vi "zc_tg.vi"(0 "action":string, 1 "LabVIEW Web Service Request":refnum<class "Web Request.lvclass"> caption="LabVIEW Web服务请求", 2 "zhriqi":string, 3 "sp_yijian":string, 4 "key":string, 5 "id":string, 7 "zc_luodi_num":string, 8 "sp_shuoming":string, 9 "didian":string, 11 "jsren":string, 13 "shuoming":string, 14 "lc_num":string) -> (15 "error":errorcluster)   [LabVIEW 2017]
uses:
  <vilib>/wsapi/Web Request.lvclass
panel:
  in  "error 3":errorcluster={"status"=TRUE, "code"=255, "source"="当前资产不是“领用”状态！"} caption="error"
  out "postdata":string caption="post数据"
  out "error out":errorcluster caption="错误输出"
  # "Web服务请求输入接线端用于调用“Web服务”选板的VI。除非不需要访问该选板，否则不要在连线板上删除这个输入接线端。"
  # "添加至连线板的每一个其他输入控件，在URL中对应于一个输入。如需在接线端模式输出（默认设置）下包含显示控件，则该显示控件必须与连线板相连。"
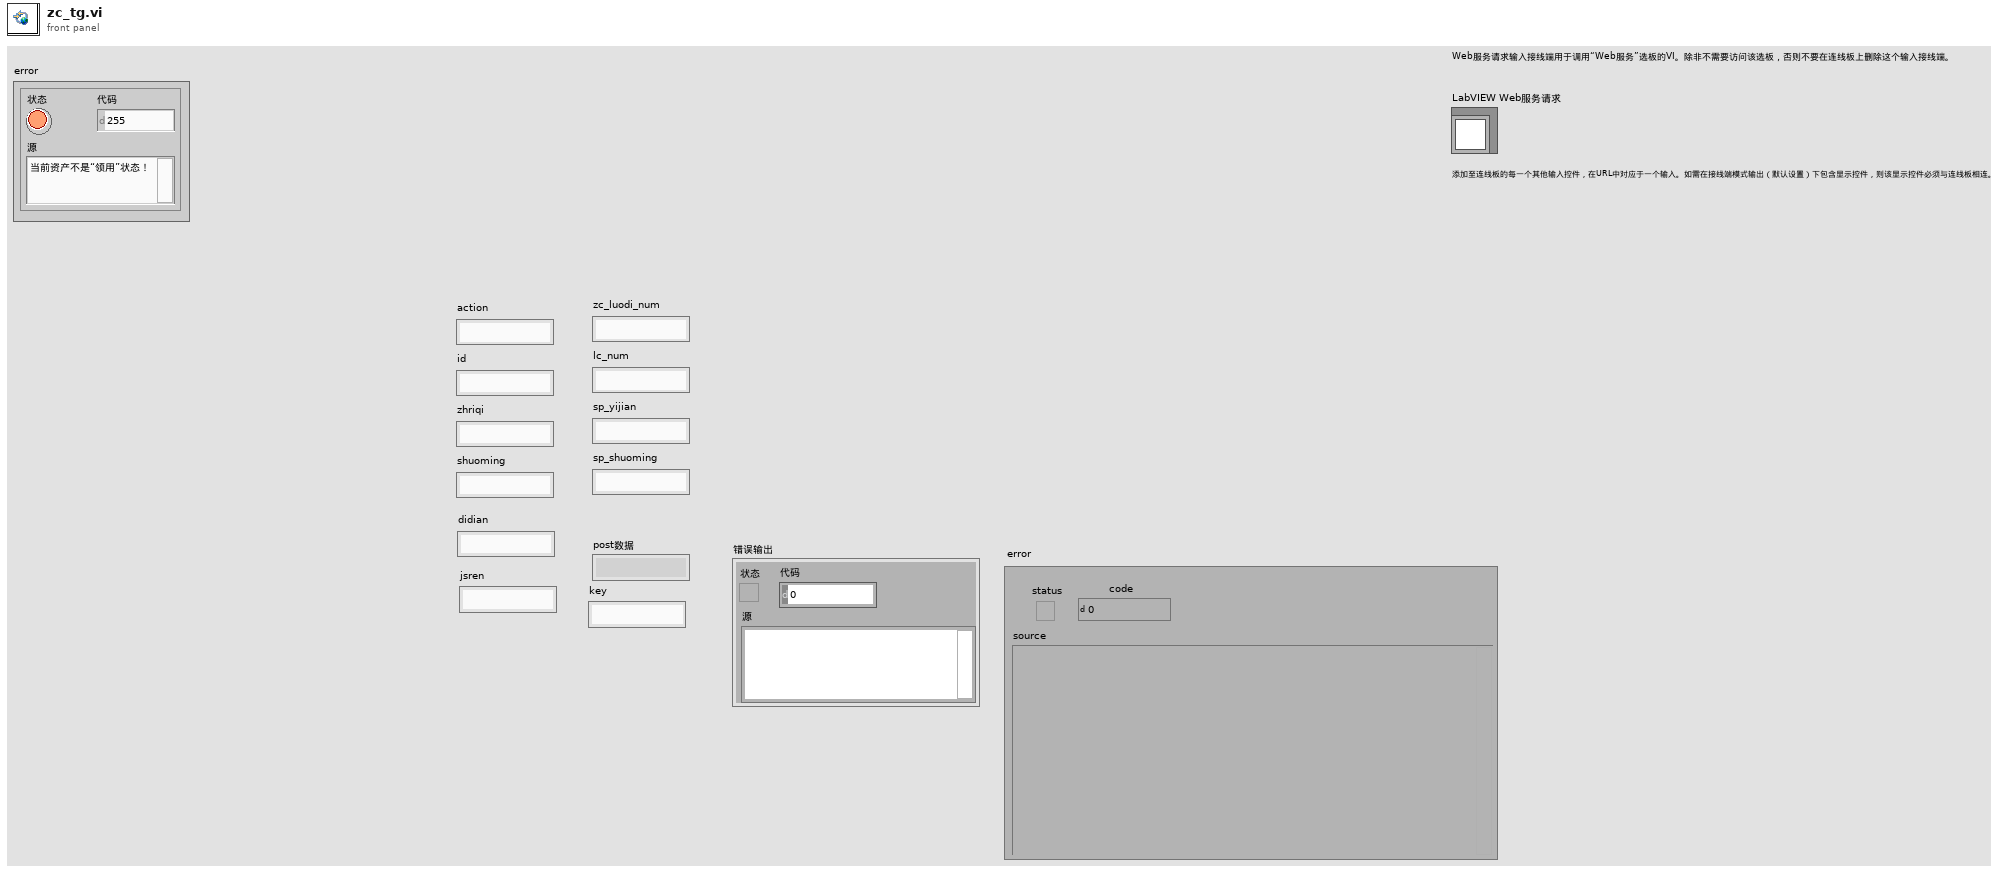
[diagram p1: front panel]
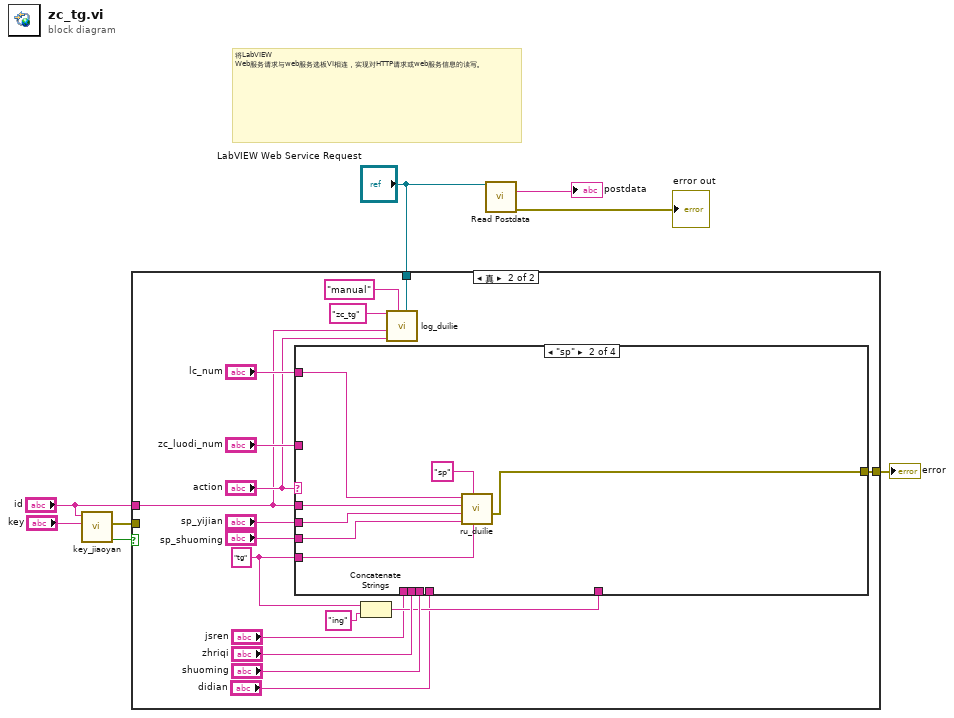
[diagram p0: block diagram]
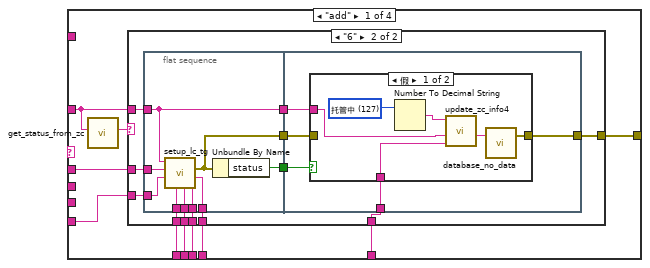
[diagram p3: hidden frame]
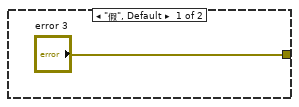
[diagram p4: hidden frame]
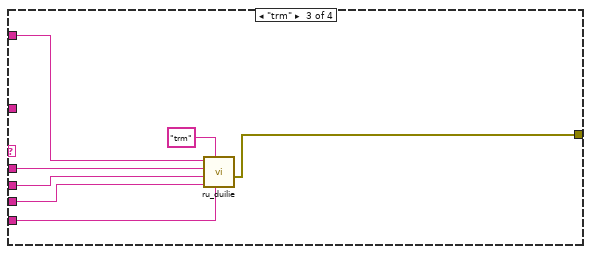
[diagram p6: hidden frame]
diagram:
  # "将LabVIEW Web服务请求与web服务选板VI相连，实现对HTTP请求或web服务信息的读写。"
  n1 = call "key_jiaoyan.vi"("key_client"="key", "gonghao"="id") -> ("jy"=w2:bool, "error"=w1:errorcluster)  [unwired: 8 in]
  n2 = case shown="真" w2 {
    tunnel: [w9 w20] -> w7
    tunnel: "LabVIEW Web Service Request" -> [_ w12]
    tunnel: "id" -> [_ w10]
    tunnel: w1 -> [w9 _]
    frame False {
    }
    frame True {
      w18 = "tg" ("yw")
      n3 = Concatenate Strings(w18, "ing" ("字符串")) -> (w17:string)
      n4 = case shown="\"sp\"" "action" {
        tunnel: w10 -> [w34 w76 w83 _]
        tunnel: "zc_luodi_num" -> [w28 _ _ _]
        tunnel: "sp_yijian" -> [_ w74 w81 _]
        tunnel: "sp_shuoming" -> [_ w73 w80 _]
        tunnel: "zhriqi" -> [w36 _ _ _]
        tunnel: "shuoming" -> [w35 _ _ _]
        tunnel: w18 -> [w33 w72 w79 _]
        tunnel: "lc_num" -> [_ w75 w82 _]
        tunnel: [w32 w71 w78 _] -> w20
        tunnel: w17 -> [w31 _ _ _]
        tunnel: "jsren" -> [w30 _ _ _]
        tunnel: "didian" -> [w29 _ _ _]
        frame "add" {
          n5 = call "get_status_from_zc.vi"("zc_luodi_num"=w28) -> ("status"=w27:string)  [unwired: 9 in, 1 out]
          n6 = case shown="\"6\"" w27 {
            tunnel: w36 -> [_ w48]
            tunnel: w35 -> [_ w47]
            tunnel: w34 -> [_ w46]
            tunnel: w33 -> [_ w45]
            tunnel: ["error 3" w44] -> w32
            tunnel: w31 -> [_ w43]
            tunnel: w30 -> [_ w42]
            tunnel: w29 -> [_ w41]
            tunnel: w28 -> [_ w40]
            frame "假", Default {
            }
            frame "6" {
              n7 = flat-sequence {
                tunnel: w48 -> [w54]
                tunnel: w47 -> [w53]
                tunnel: w40 -> [w58]
                tunnel: w46 -> [w56]
                tunnel: w45 -> [w57]
                tunnel: [w58] -> w49
                tunnel: w42 -> [w55]
                tunnel: w41 -> [w52]
                tunnel: [w51] -> w39
                tunnel: [w50] -> w38
                tunnel: w49 -> [w62]
                tunnel: [w63] -> w44
                tunnel: w43 -> [w61]
                tunnel: w39 -> [w60]
                tunnel: w38 -> [w59]
                frame #0 {
                  n8 = call "setup_lc_tg.vi"("shuoming"=w53, "didian"=w52, "zhriqi"=w54, "jsren"=w55, "yw"=w57, "id"=w56, "zc_luodi_num"=w58) -> ("error"=w50:errorcluster)  [unwired: 4 in]
                  n9 = Unbundle By Name(w50) -> ("status"=w51:bool)
                }
                frame #1 {
                  n10 = case shown="假" w60 {
                    tunnel: [w68 w70] -> w63
                    tunnel: w62 -> [w66 _]
                    tunnel: w61 -> [w65 _]
                    tunnel: w59 -> [_ w70]
                    frame False {
                      w67 = u8 127 items=["待验收"=1, "无需验收"=2, "验收不合格"=3, "待入库"=4, "入库"=5, "领用"=6, "借用"=7, "托管"=8, "接管"=9, "退出"=10, "出库在用"=11, "盘亏"=12, "出售"=13, "报废"=14, "领用中"=120, "退库中"=121, "借用中"=122, "归还中"=123, "转移中"=124, "调拨中"=125, "借调中"=126, "托管中"=127, "终止托管中"=128, "退出中"=129, "处置中"=130] ("状态选择器")
                      n11 = Number To Decimal String(number=w67) -> (decimal integer string=w64:string)  [unwired: 1 in]
                      n12 = call "update_zc_info4.vi"("ywxinxi"=w65, "number"=w66, "status"=w64) -> ("data_str"=w69:string)  [unwired: 8 in]
                      n13 = call "database_no_data.vi"("input"=w69) -> ("error"=w68:errorcluster)  [unwired: 2 in]
                    }
                    frame True {
                    }
                  }
                }
              }
            }
          }
        }
        frame "sp" {
          n14 = call "ru_duilie.vi"("yw"=w72, "name"="sp" ("元素"), "sp_shuoming"=w73, "sp_yijian"=w74, "id"=w76, "lc_num"=w75) -> ("error"=w71:errorcluster)  [unwired: 5 in]
        }
        frame "trm" {
          n15 = call "ru_duilie.vi"("yw"=w79, "name"="trm" ("元素"), "sp_shuoming"=w80, "sp_yijian"=w81, "id"=w83, "lc_num"=w82) -> ("error"=w78:errorcluster)  [unwired: 5 in]
        }
        frame Default {
        }
      }
      n16 = call "log_duilie.vi"("LabVIEW Web Service Request"=w12, "type"="manual", "action"="action", "user"=w10, "yw"="zc_tg") -> ()  [unwired: 7 in]
    }
  }
  "error" <- w7
  n17 = call <vilib>:"Read Postdata.vi"("LabVIEW Web Service Request"="LabVIEW Web Service Request") -> ("postdata"=→"postdata":string, "error out"=→"error out":errorcluster)  [unwired: 12 in, 1 out]
